vi "PrechargeState.vi"(8 "error in (no error)":errorcluster, 9 "Cluster in":T2, 10 "Enum in":T1, 11 "Actual Start [i]":i64) -> (0 "error out":errorcluster, 2 "Cluster out":T2, 3 "Enum":T1)   [LabVIEW 2018]
uses:
  Type_Def Actuator Controls.ctl
  Type_Def_ControlState.ctl
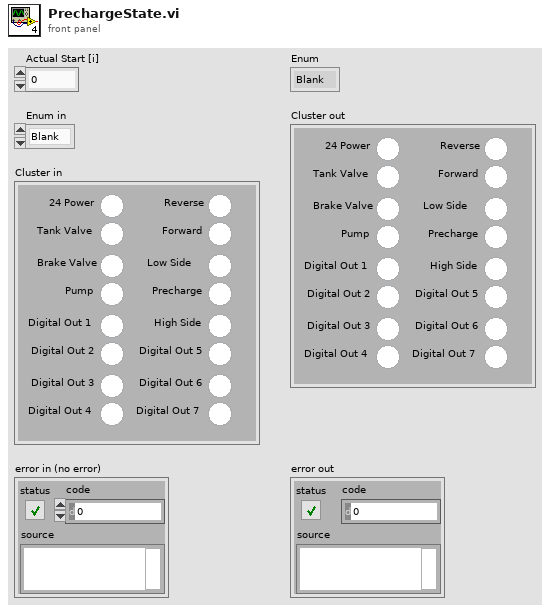
[diagram p1: front panel]
types:
  T1 = typedef "Type_Def_ControlState.ctl" = enum16{"Blank", "Systems Check", "Idle", "Ready", "Pushing", "CrawlingPrecharge", "Braking", "Fault", "Boot Up", "Unpowered", "Crawling", "Shutdown", "Service Push", "Service Wait", "Vent", "Precharge", "Cooldown"}
  T2 = typedef "Type_Def Actuator Controls.ctl" = cluster{"Reverse ":bool, "Forward":bool, "Low Side":bool, "Precharge":bool, "High Side":bool, "Digital Out 5":bool, "Digital Out 6":bool, "Digital Out 7 ":bool, "24 Power":bool, "Tank Valve ":bool, "Brake Valve":bool, "Pump":bool, "Digital Out 1 ":bool, "Digital Out 2":bool, "Digital Out 3":bool, "Digital Out 4 ":bool}
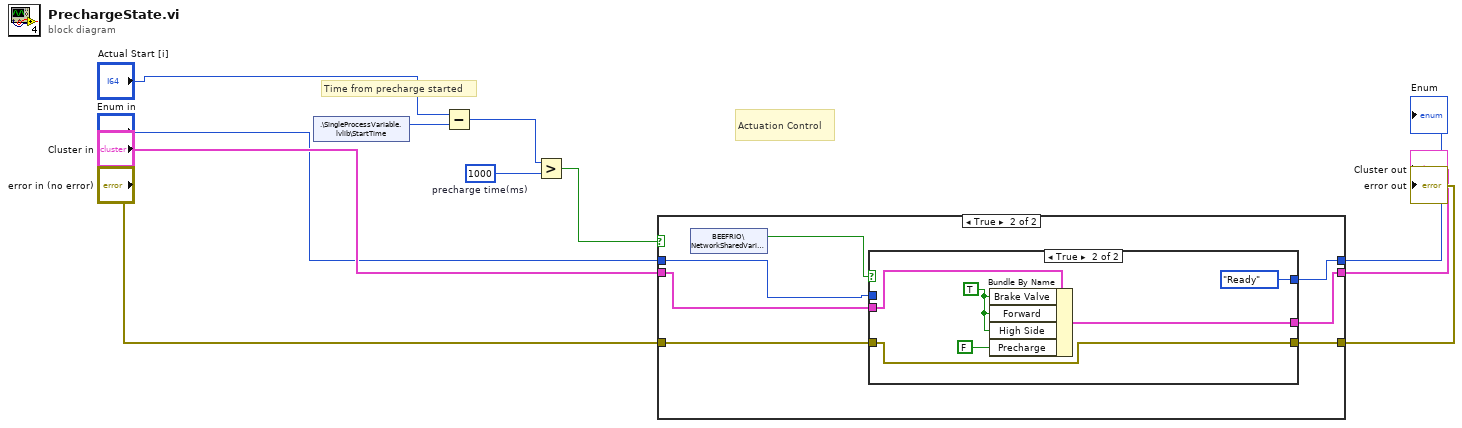
[diagram p0: block diagram]
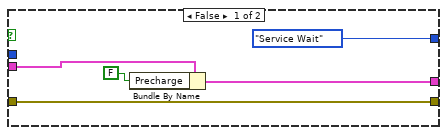
[diagram p3: hidden frame]
diagram:
  w10 = i64 1000  # precharge time(ms)
  # "Time from precharge started"
  # "Actuation Control"
  n1 = shared-variable ".\\SingleProcessVariable.lvlib\\StartTime"() -> (w8:i64)  [unwired: 1 in, 1 out]
  n2 = Subtract(x="Actual Start [i]", y=w8) -> (x-y=w9:i64)
  n3 = Greater?(x=w9, y=w10) -> (0:w11:bool)
  n4 = case shown="True" w11 {
    tunnel: "Enum in" -> [w14 w21]
    tunnel: [w14 w20] -> w2
    tunnel: "Cluster in" -> [w13 w19]
    tunnel: [w13 w18] -> w4
    tunnel: [w12 w17] -> w5
    tunnel: "error in (no error)" -> [w12 w16]
    frame False {
    }
    frame True {
      n5 = shared-variable "BEEFRIO\\NetworkSharedVariable.lvlib\\Ready"() -> (w15:bool)  [unwired: 1 in, 1 out]
      n6 = case shown="True" w15 {
        tunnel: w21 -> [_ _]
        tunnel: [Type_Def_ControlState."Service Wait" Type_Def_ControlState."Ready"] -> w20
        tunnel: w19 -> [w24 w31]
        tunnel: [w23 w30] -> w18
        tunnel: [w26 w29] -> w17
        tunnel: w16 -> [w26 w29]
        frame False {
          n7 = Bundle By Name(cluster=w24, "Precharge"=FALSE) -> (w23:T2)
        }
        frame True {
          w28 = TRUE
          n8 = Bundle By Name(cluster=w31, "Brake Valve"=w28, "Forward"=w28, "High Side"=w28, "Precharge"=FALSE) -> (w30:T2)
        }
      }
    }
  }
  "error out" <- w5
  "Cluster out" <- w4
  "Enum" <- w2
